vi "App - RUS scan.vi"(0 "Lock-in DAQ settings":T5={"Lockin mode"=enum."NI-DAQ", "DAQmx Device"="Dev1", "SR Lockin"="GPIB0::10::INSTR", "Clock Multiplier"=64, "Low-pass filter"=enum."No filtering", "Ranges and couplings "=[{"Range"=2.5, "Coupling"=10106}], "Samples per read"=20, "Record IF"=FALSE, "Auto-phase"=FALSE, "RP IP Addres"="172.20.117.190"} {"Ranges and couplings"."Coupling" items=["default"=-1, "RSE"=10083, "NRSE"=10078, "Differential"=10106, "Pseudodifferential"=12529]}, 1 "Save data settings":T7={"Save data"=TRUE, "Data Root Path"=path "E:/Technique/RUS/Saphire/Saphire_piece1/1_test", "File Prefix"="291.30300K_2000_3000_2.00000V_0.00000T_Jul26-2016__14-58-15_", "File Format"=enum."BINARY", "Save column names"=FALSE, "File Comments"="\r\nColumns:Frequency\\tX\\tY\r\n    ITC Temp= 299.200000\r\n    LTC Temp= 0.000000\r\n          ITC_set=295.00000\r\n", "User/Prj"="<User Name/Project Description>"}, 5 "temperature":dbl=291.303, 7 "sweep settings":T1={"time gap (min) "=0.0, "Bypass error dialog"=TRUE, "range factor"=1.2, "min gamma(kHz)"=0.005, "max step(Hz)"=1500.0, "min step(Hz)"=0.001, "save freq units"=enum."kHz", "Zero signal?"=FALSE, "time in Gamma --OK"=FALSE, "scan mode"=enum."uniform", "power control mode "=enum."none", "time-in-gamma mode"=enum."uniform scan"}, 9 "Fast swep settings":T4={"Update rate (Hz)"=200.0, "Start F, Hz"=2000000.0, "Stop F"=3000000.0, "Number of points"=5760, "Amplitude"=2.0, "Init&amplitude"=TRUE, "IF"=1000.0, "Time constant"=0.0042} {"IF" format="%#_6p"; "Amplitude" min=0.0 max=2.5; "Number of points" format="%.0p"; "Stop F" format="%#_6p"; "Start F, Hz" format="%#_6p"; "Update rate (Hz)" format="%0.2f"}, 11 "error in (no error)":errorcluster) -> (6 "Actual file path":path=path "E:/Technique/RUS/Saphire/Saphire_piece1/1_test/July_2016/072616/291.31700K_2000_3000_2.00000V_0.00000T_Jul26-2016__14-57-42_001_072616.bin", 15 "error out":errorcluster)   [LabVIEW 2016]
uses:
  <vilib>/Utility/error.llb/DialogType.ctl
  <resource>/objmgr/daqmx.rc
  next chunk -- action.ctl
  cursor action.ctl
  four-corner circle transformation.ctl
  circle corners.ctl
  NHMFL_Core/Libraries/Red Pitaya/RP Core/RP Transceiver/RP Transceiver.lvclass
  resonant_ultrasound/Libraries/RUS/Controls/Sweep settings.ctl
  resonant_ultrasound/Libraries/RUS/Controls/Lock-in DAQ settings.ctl
  NHMFL_Core/Libraries/File/Controls/File formats.ctl
  NHMFL_Core/Libraries/File/Controls/Save data settings.ctl
  single sweep - adaptive parameters.ctl
  single sweep - frequency chunks.ctl
  wavepacket.ctl
  next chunk -- parameters.ctl
  next chunk -- algorithm.ctl
  find peak -- parameters.ctl
  adaptive sweep UI controls.ctl
  time in gamma mode control.ctl
  resonant_ultrasound/Libraries/RUS/Controls/Lockin mode.ctl
panel:
  in  "Tab : everything":enum32{"main", "everything else", "adaptive"}(tab)
  out "near omega (kHz)":dbl
  in  "Subtract a circle?":enum16{"Yes", "No"}(ring)=enum."No"
  in  "complex plane scale gauge":dbl(slide)=0.012396748308571648 caption="Volts" scale=0.0001..0.5
  in  "show plot pallets":bool=TRUE
  in  "highlight last # sec":dbl=5.0
  out "Plot:response":cluster{dbl[], dbl[]}[](graph)=[{array[5760 elements], array[960 elements]}, {array[5760 elements], array[960 elements]}, {[2225.33441, 2225.33441], [-0.001, 0.001]}, {[3002.8544, 3002.8544], [-0.001, 0.001]}, {[4313.39901, 4313.39901], [-0.001, 0.001]}, {[4368.99077, 4368.99077], [-0.001, 0.001]}, {[5103.78232, 5103.78232], [-0.001, 0.001]}, {[5322.11972, 5322.11972], [-0.001, 0.001]}, {[5780.98612, 5780.98612], [-0.001, 0.001]}, {[6352.47126, 6352.47126], [-0.001, 0.001]}]
  out "Plot:complex plane":cluster{dbl[], dbl[]}[](graph)=[{array[960 elements], array[960 elements]}, {array[1000 elements], array[1000 elements]}, {[0.005000003045536789, 0.004940547817909086, 0.004763119779482496, 0.004470517076413378, 0.004067354228121515, 0.0035599893535622827, 0.0029564238998925634, 0.0022661764548692546, 0.0015001326330342118, 0.0006703734030701707, -0.00021001543629219814, -0.0011271496271373508, -0.0020665654154062474, -0.003013447652938098, -0.003952863441206996, -0.004869997632052148, -0.005750386471414516, -0.0065801457013785584, -0.0073461895232136, -0.008036436968236908, -0.008640002421906627, -0.009147367296465859, -0.009550530144757723, -0.00984313284782684, -0.010020560886253431, -0.010080016113881134, -0.010020560886253431, -0.00984313284782684, -0.009550530144757721, -0.009147367296465859, -0.008640002421906625, -0.008036436968236908, -0.007346189523213599, -0.006580145701378555, -0.005750386471414511, -0.004869997632052148, -0.003952863441206995, -0.0030134476529380966, -0.0020665654154062444, -0.0011271496271373462, -0.00021001543629219988, 0.0006703734030701703, 0.0015001326330342135, 0.0022661764548692572, 0.002956423899892566, 0.0035599893535622853, 0.004067354228121515, 0.004470517076413378, 0.004763119779482496, 0.004940547817909086], [0.00047076259399639255, 0.0014157763757271474, 0.0023458867255961384, 0.0032464252477649408, 0.004103189911783316, 0.004902669027093289, 0.0056322543304607505, 0.00628043982581846, 0.006837003240697381, 0.007293167237570003, 0.007641737837706482, 0.007877217874516685, 0.007995893687151154, 0.007995893687151154, 0.007877217874516684, 0.007641737837706482, 0.0072931672375700024, 0.00683700324069738, 0.00628043982581846, 0.005632254330460749, 0.0049026690270932895, 0.004103189911783315, 0.003246425247764939, 0.002345886725596139, 0.0014157763757271461, 0.0004707625939963901, -0.00047425118773436253, -0.0014043615376033549, -0.0023049000597721585, -0.0031616647237905308, -0.0039611438391005055, -0.004690729142467966, -0.005338914637825676, -0.005895478052704598, -0.00635164204957722, -0.0067002126497136974, -0.0069356926865239, -0.007054368499158369, -0.007054368499158369, -0.006935692686523899, -0.006700212649713698, -0.006351642049577218, -0.005895478052704595, -0.0053389146378256735, -0.004690729142467962, -0.0039611438391004995, -0.0031616647237905303, -0.002304900059772155, -0.001404361537603351, -0.00047425118773435874]}, {[-0.0036773228927567273, -0.003563591256898272, -0.0034498596210398164, -0.003336127985181361, -0.0032223963493229054, -0.0031086647134644495, -0.0029949330776059945, -0.0028812014417475386, -0.002767469805889083, -0.0026537381700306277, -0.0025400065341721722, -0.0024262748983137168, -0.0023125432624552613, -0.002198811626596806, -0.00208507999073835, -0.001971348354879895, -0.0018576167190214393, -0.0017438850831629838, -0.0016301534473045281, -0.0015164218114460727], [0.00792450366560593, 0.007179129558444975, 0.006433755451284022, 0.005688381344123069, 0.004943007236962115, 0.004197633129801161, 0.0034522590226402083, 0.0027068849154792546, 0.001961510808318301, 0.001216136701157347, 0.0004707625939963933, -0.00027461151316456045, -0.0010199856203255125, -0.0017653597274864662, -0.00251073383464742, -0.0032561079418083737, -0.0040014820489693275, -0.004746856156130281, -0.005492230263291235, -0.006237604370452189]}, {[0.004913734537437363, 0.004168360430276409, 0.003422986323115456, 0.0026776122159545028, 0.001932238108793549, 0.0011868640016325952, 0.00044148989447164236, -0.0003038842126893114, -0.0010492583198502652, -0.001794632427011219, -0.0025400065341721727, -0.0032853806413331264, -0.0040307547484940785, -0.004776128855655032, -0.005521502962815986, -0.00626687706997694, -0.0070122511771378935, -0.007757625284298847, -0.008502999391459801, -0.009248373498620755], [0.0016080789525809475, 0.001494347316722492, 0.0013806156808640366, 0.001266884045005581, 0.0011531524091471254, 0.00103942077328867, 0.0009256891374302145, 0.0008119575015717589, 0.0006982258657133035, 0.0005844942298548479, 0.00047076259399639244, 0.000357030958137937, 0.00024329932227948152, 0.00012956768642102606, 1.5836050562570382e-05, -9.789558529588508e-05, -0.00021162722115434054, -0.000325358857012796, -0.0004390904928712517, -0.0005528221287297071]}]
  in  "progress (sec)":dbl(slide)=4.701000000000931 caption="seconds" min=80.0 max=80.0 scale=0.0..28.8
  in  "Plot when running":bool=TRUE
  in  "Graph update rate, ms":u32=50
  out "near gamma (kHz)":dbl
  in  "stop":bool
  out "Progress, %":u8(slide)=16 scale=0.0..100.0
  in  "Tab : sweep controls":enum32{"Main controls", "File", "Advanced"}(tab)
  in  "Manual\nPhase":dbl(slide) scale=-180.0..180.0
  out "Error status byte\n(bit 5 - FAST aborted)":u8 format="%08b"
  out "STD status byte":u8 format="%08b"
  out "DO array  making time":u32
  out "DO write time, ms":u32=37
  out "Loop counter":i32=287
  out "Pre-sweep delay, s":dbl=0.2
  out "Samples in buffer":u32
  out "Actual setup time, ms":u32=2842
  out "line two":cluster{dbl[], dbl[]}={[0.004913734537437363, 0.004168360430276409, 0.003422986323115456, 0.0026776122159545028, 0.001932238108793549, 0.0011868640016325952, 0.00044148989447164236, -0.0003038842126893114, -0.0010492583198502652, -0.001794632427011219, -0.0025400065341721727, -0.0032853806413331264, -0.0040307547484940785, -0.004776128855655032, -0.005521502962815986, -0.00626687706997694, -0.0070122511771378935, -0.007757625284298847, -0.008502999391459801, -0.009248373498620755], [0.0016080789525809475, 0.001494347316722492, 0.0013806156808640366, 0.001266884045005581, 0.0011531524091471254, 0.00103942077328867, 0.0009256891374302145, 0.0008119575015717589, 0.0006982258657133035, 0.0005844942298548479, 0.00047076259399639244, 0.000357030958137937, 0.00024329932227948152, 0.00012956768642102606, 1.5836050562570382e-05, -9.789558529588508e-05, -0.00021162722115434054, -0.000325358857012796, -0.0004390904928712517, -0.0005528221287297071]}
  out "circle":cluster{dbl[], dbl[]}={[0.005000003045536789, 0.004940547817909086, 0.004763119779482496, 0.004470517076413378, 0.004067354228121515, 0.0035599893535622827, 0.0029564238998925634, 0.0022661764548692546, 0.0015001326330342118, 0.0006703734030701707, -0.00021001543629219814, -0.0011271496271373508, -0.0020665654154062474, -0.003013447652938098, -0.003952863441206996, -0.004869997632052148, -0.005750386471414516, -0.0065801457013785584, -0.0073461895232136, -0.008036436968236908, -0.008640002421906627, -0.009147367296465859, -0.009550530144757723, -0.00984313284782684, -0.010020560886253431, -0.010080016113881134, -0.010020560886253431, -0.00984313284782684, -0.009550530144757721, -0.009147367296465859, -0.008640002421906625, -0.008036436968236908, -0.007346189523213599, -0.006580145701378555, -0.005750386471414511, -0.004869997632052148, -0.003952863441206995, -0.0030134476529380966, -0.0020665654154062444, -0.0011271496271373462, -0.00021001543629219988, 0.0006703734030701703, 0.0015001326330342135, 0.0022661764548692572, 0.002956423899892566, 0.0035599893535622853, 0.004067354228121515, 0.004470517076413378, 0.004763119779482496, 0.004940547817909086], [0.00047076259399639255, 0.0014157763757271474, 0.0023458867255961384, 0.0032464252477649408, 0.004103189911783316, 0.004902669027093289, 0.0056322543304607505, 0.00628043982581846, 0.006837003240697381, 0.007293167237570003, 0.007641737837706482, 0.007877217874516685, 0.007995893687151154, 0.007995893687151154, 0.007877217874516684, 0.007641737837706482, 0.0072931672375700024, 0.00683700324069738, 0.00628043982581846, 0.005632254330460749, 0.0049026690270932895, 0.004103189911783315, 0.003246425247764939, 0.002345886725596139, 0.0014157763757271461, 0.0004707625939963901, -0.00047425118773436253, -0.0014043615376033549, -0.0023049000597721585, -0.0031616647237905308, -0.0039611438391005055, -0.004690729142467966, -0.005338914637825676, -0.005895478052704598, -0.00635164204957722, -0.0067002126497136974, -0.0069356926865239, -0.007054368499158369, -0.007054368499158369, -0.006935692686523899, -0.006700212649713698, -0.006351642049577218, -0.005895478052704595, -0.0053389146378256735, -0.004690729142467962, -0.0039611438391004995, -0.0031616647237905303, -0.002304900059772155, -0.001404361537603351, -0.00047425118773435874]}
  out "line one":cluster{dbl[], dbl[]}={[-0.0036773228927567273, -0.003563591256898272, -0.0034498596210398164, -0.003336127985181361, -0.0032223963493229054, -0.0031086647134644495, -0.0029949330776059945, -0.0028812014417475386, -0.002767469805889083, -0.0026537381700306277, -0.0025400065341721722, -0.0024262748983137168, -0.0023125432624552613, -0.002198811626596806, -0.00208507999073835, -0.001971348354879895, -0.0018576167190214393, -0.0017438850831629838, -0.0016301534473045281, -0.0015164218114460727], [0.00792450366560593, 0.007179129558444975, 0.006433755451284022, 0.005688381344123069, 0.004943007236962115, 0.004197633129801161, 0.0034522590226402083, 0.0027068849154792546, 0.001961510808318301, 0.001216136701157347, 0.0004707625939963933, -0.00027461151316456045, -0.0010199856203255125, -0.0017653597274864662, -0.00251073383464742, -0.0032561079418083737, -0.0040014820489693275, -0.004746856156130281, -0.005492230263291235, -0.006237604370452189]}
  out "frequency":dbl[](array[numeric])
  out "complex data":cdb[](array[numeric])
  out "#data points so far":i32=960
  out "last data":cdb[](array[numeric])=[-1.8863502679099892e-05+1.1101912486449137e-05i, -1.3771240984552797e-05+1.353770104896233e-05i, 8.815893688967333e-06-8.669622050274321e-07i, 4.353149549589407e-06-5.242292389749474e-06i, -2.0188892981734304e-05+2.69270732421671e-06i, -3.236472954490424e-05-1.4037098105498458e-05i, -1.4486448565831475e-06+5.6829496403972965e-06i, 2.1749189330097788e-05-2.2323271152381018e-05i, 1.0947860915724242e-05-9.35400417253664e-06i, 1.002480840777342e-06+1.0320450470074709e-05i, 1.7405541793727768e-05+1.8150037416439624e-05i, -3.440648475476081e-06-3.0319378431607727e-06i, -5.515652282118088e-06+8.369787998015825e-06i, 1.3508753228977962e-06-9.402754381312778e-07i, -9.163410786339015e-06+3.1872150390602785e-05i, 1.843763405159508e-05+9.77165232492216e-07i, 1.6194427097054223e-05+8.11657185157076e-06i, -1.892640018440827e-05+1.3227915471368098e-05i, -1.8081522602619296e-05+1.6532235062315973e-05i, 1.084682936928357e-05+3.944687906764937e-06i]
  out "fancy circles":cluster{dbl[], dbl[]}[](array[cluster])
  out "fancy lines":cluster{dbl[], dbl[]}[](array[cluster])=[{[2225.33441, 2225.33441], [-0.001, 0.001]}, {[3002.8544, 3002.8544], [-0.001, 0.001]}, {[4313.39901, 4313.39901], [-0.001, 0.001]}, {[4368.99077, 4368.99077], [-0.001, 0.001]}, {[5103.78232, 5103.78232], [-0.001, 0.001]}, {[5322.11972, 5322.11972], [-0.001, 0.001]}, {[5780.98612, 5780.98612], [-0.001, 0.001]}, {[6352.47126, 6352.47126], [-0.001, 0.001]}]
  in  "adaptive state":T9={"peaks are known -- parameters"={"Def Gamma (kHz)"=10.0, "dV"=17.0, "time in Gamma (sec)"=3.0, "phi-star"=0.0, "all peaks (kHz)"=[2225.33441, 3002.8544, 4313.39901, 4368.99077, 5103.78232, 5322.11972, 5780.98612, 6352.47126], "delta t (sec)"=0.005, "default step (Hz)"=173.61111111111111, "all gamma (kHz)"=[0.92069, 0.9684, 1.01783, 0.32516, 1.96607, 0.61241, 0.19018, 0.73869], "peaks OK"=TRUE, "gamma OK"=TRUE, "near omega (kHz)"=0.0, "near gamma (kHz)"=0.0, "min step (Hz)"=0.001, "max step(Hz)"=1500.0, "min gamma (kHz)"=0.005, "all time in gamma (sec)"=[], "time in gamma OK"=FALSE, "time-in-gamma mode"=enum."same for all"}, "find peak - parameters"={"wavepacket"={"R"=0.5, "wave number"=17.0, "delta k"=7.0, "radii vector"=[], "radial section"=[], "wave vector"=22.0, "wavepacket is"=TRUE}, "number of grid points"=70, "decimation threshold"=1, "Voltage range"=0.1, "target freq step"=20.0, "target spot size"=0.05, "factor"=1.0, "another factor"=1.0, "analyze last # sec"=3, "scale factor"=3}} {"find peak - parameters"."wavepacket"."delta k" format="%#_3f"; "find peak - parameters"."wavepacket"."wave number" format="%#_3f"; "find peak - parameters"."wavepacket"."R" format="%#_3f"}
  in  "chunks":T13={"start F (Hz)"=2000000.0, "stop F (Hz)"=3000000.0, "total number of points"=5760, "chunk size"=20, "freq step (Hz)"=173.61111111111111, "update rate (Hz)"=200.0, "adaptive parameters"={"peaks are known -- parameters"={"Def Gamma (kHz)"=10.0, "dV"=17.0, "time in Gamma (sec)"=3.0, "phi-star"=0.0, "all peaks (kHz)"=[2225.33441, 3002.8544, 4313.39901, 4368.99077, 5103.78232, 5322.11972, 5780.98612, 6352.47126], "delta t (sec)"=0.005, "default step (Hz)"=173.61111111111111, "all gamma (kHz)"=[0.92069, 0.9684, 1.01783, 0.32516, 1.96607, 0.61241, 0.19018, 0.73869], "peaks OK"=TRUE, "gamma OK"=TRUE, "near omega (kHz)"=0.0, "near gamma (kHz)"=0.0, "min step (Hz)"=0.001, "max step(Hz)"=1500.0, "min gamma (kHz)"=0.005, "all time in gamma (sec)"=[], "time in gamma OK"=FALSE, "time-in-gamma mode"=enum."same for all"}, "find peak - parameters"={"wavepacket"={"R"=0.5, "wave number"=17.0, "delta k"=7.0, "radii vector"=[], "radial section"=[], "wave vector"=22.0, "wavepacket is"=TRUE}, "number of grid points"=70, "decimation threshold"=1, "Voltage range"=0.1, "target freq step"=20.0, "target spot size"=0.05, "factor"=1.0, "another factor"=1.0, "analyze last # sec"=3, "scale factor"=3}}, "total sweep time (sec)"=28.8, "chunk time (sec)"=0.1, "spot size (V)"=0.0, "uniform freq step (Hz)"=173.61111111111111, "next start freq (Hz)"=2177083.3333333293} {"next start freq (Hz)" format="%#9_8f"; "uniform freq step (Hz)" format="%#_3f"; "spot size (V)" format="%#_2f"; "adaptive parameters"."find peak - parameters"."wavepacket"."delta k" format="%#_3f"; "adaptive parameters"."find peak - parameters"."wavepacket"."wave number" format="%#_3f"; "adaptive parameters"."find peak - parameters"."wavepacket"."R" format="%#_3f"; "freq step (Hz)" format="%#4_4f"; "stop F (Hz)" format="%#_3f"; "start F (Hz)" format="%#_3f"}
  # "SRS Lockin related"
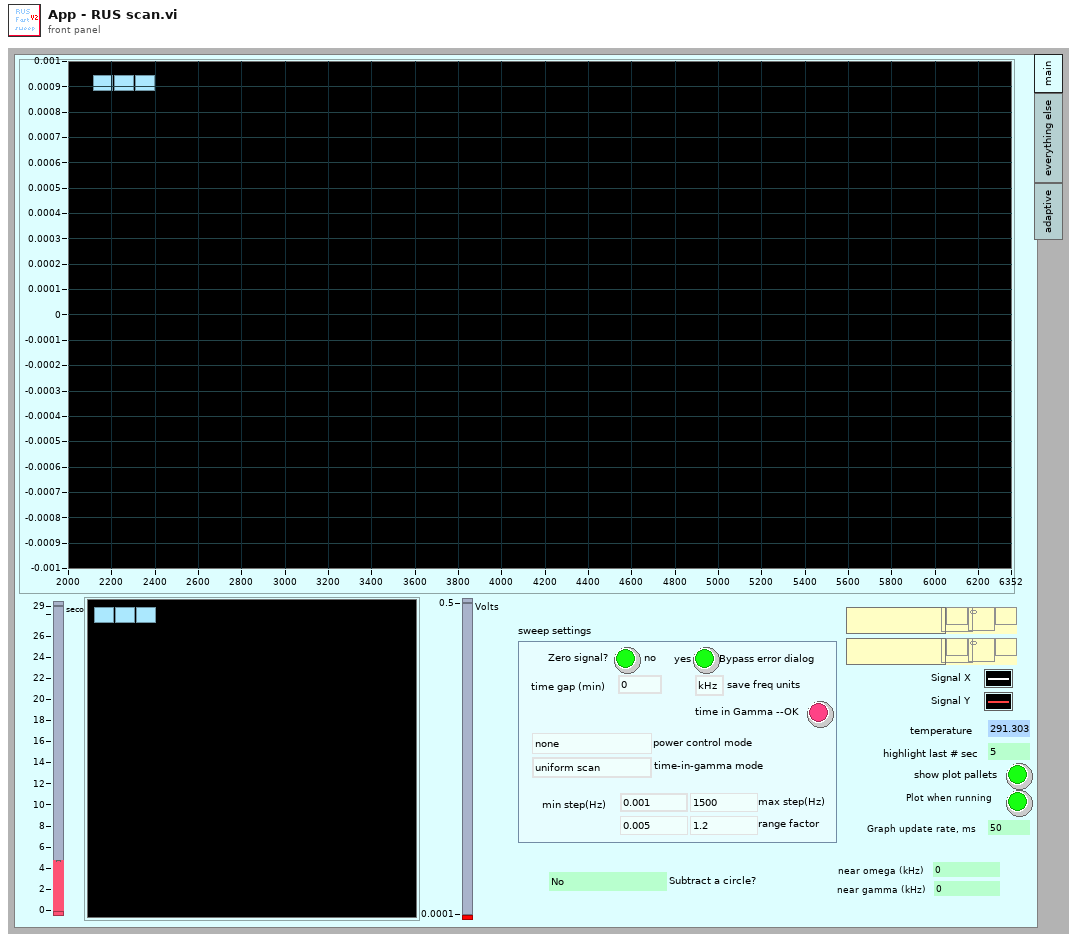
[diagram p1: front panel]
types:
  T1 = typedef "adaptive sweep UI controls.ctl" = cluster{"time gap (min) ":dbl, "Bypass error dialog":bool, "range factor":dbl, "min gamma(kHz)":dbl, "max step(Hz)":dbl, "min step(Hz)":dbl, "save freq units":enum16{"kHz", "Hz"}, "Zero signal?":bool, "time in Gamma --OK":bool, "scan mode":T2, "power control mode ":enum16{"power vs Temp", "power vs Time", "none"}, "time-in-gamma mode":T3}
  T2 = typedef "next chunk -- algorithm.ctl" = enum16{"peak position is known", "uniform", "predictive"}
  T3 = typedef "time in gamma mode control.ctl" = enum16{"same for all", "each one different", "uniform scan"}
  T4 = typedef "Sweep settings.ctl" = cluster{"Update rate (Hz)":dbl, "Start F, Hz":dbl, "Stop F":dbl, "Number of points":i32, "Amplitude":dbl, "Init&amplitude":bool, "IF":dbl, "Time constant":dbl}
  T5 = typedef "Lock-in DAQ settings.ctl" = cluster{"Lockin mode":T6, "DAQmx Device":tag, "SR Lockin":refnum<visa-resource-name>, "Clock Multiplier":i32, "Low-pass filter":enum16{"No filtering", "Butterworth", "Bessel"}, "Ranges and couplings ":cluster{"Range":dbl, "Coupling":i32}[], "Samples per read":i32, "Record IF":bool, "Auto-phase":bool, "RP IP Addres":string}
  T6 = typedef "Lockin mode.ctl" = enum16{"SRS", "NI-DAQ", "Pitaya"}
  T7 = typedef "Save data settings.ctl" = cluster{"Save data":bool, "Data Root Path":path, "File Prefix":string, "File Format":T8, "Save column names":bool, "File Comments":string, "User/Prj":string}
  T8 = typedef "File formats.ctl" = enum16{"TDMS", "ASCII", "BINARY"}
  T9 = typedef "single sweep - adaptive parameters.ctl" = cluster{"peaks are known -- parameters":T10, "find peak - parameters":T11}
  T10 = typedef "next chunk -- parameters.ctl" = cluster{"Def Gamma (kHz)":dbl, "dV":dbl, "time in Gamma (sec)":dbl, "phi-star":dbl, "all peaks (kHz)":dbl[], "delta t (sec)":dbl, "default step (Hz)":dbl, "all gamma (kHz)":dbl[], "peaks OK":bool, "gamma OK":bool, "near omega (kHz)":dbl, "near gamma (kHz)":dbl, "min step (Hz)":dbl, "max step(Hz)":dbl, "min gamma (kHz)":dbl, "all time in gamma (sec)":dbl[], "time in gamma OK":bool, "time-in-gamma mode":T3}
  T11 = typedef "find peak -- parameters.ctl" = cluster{"wavepacket":T12, "number of grid points":i32, "decimation threshold":i32, "Voltage range":dbl, "target freq step":dbl, "target spot size":dbl, "factor":dbl, "another factor":dbl, "analyze last # sec":i32, "scale factor":i32}
  T12 = typedef "wavepacket.ctl" = cluster{"R":dbl, "wave number":dbl, "delta k":dbl, "radii vector":dbl[], "radial section":cdb[], "wave vector":dbl, "wavepacket is":bool}
  T13 = typedef "single sweep - frequency chunks.ctl" = cluster{"start F (Hz)":dbl, "stop F (Hz)":dbl, "total number of points":i32, "chunk size":i32, "freq step (Hz)":dbl, "update rate (Hz)":dbl, "adaptive parameters":T9, "total sweep time (sec)":dbl, "chunk time (sec)":dbl, "spot size (V)":dbl, "uniform freq step (Hz)":dbl, "next start freq (Hz)":dbl}
  T14 = typedef "RUS settings.ctl" = cluster{"NI-DAQ lockin settings":T15, "Fast swep settings":T4, "Pre-sweep delay, s":dbl, "Lockin mode":T6, "SR Lockin":refnum<visa-resource-name>, "DAQmx Device":tag, "Clock Multiplier":i32, "Fast Sweep Data Out":cluster{"DO clock task":refnum<k21>, "DO task":refnum<k21>, "Update clock task":refnum<k21>, "DAQ lockin task":refnum<k21>, "Pre-sweep counter task":refnum<k21>}, "Lockin Range, V":sgl, "F Array":dbl[], "Freq. update clock terminal":string, "DO Clock Rate (Hz)":dbl, "ADC clock terminal":string, "Pre-sweep counter terminal":string, "Samples per read":i32, "DO clock terminal":string, "Pre-sweep points":i32, "F points per write":i32, "Total sweep time, s":dbl, "Initial SYNTH phase":dbl, "Record IF":bool, "Save data settings":T7, "Data file path":path, "New data user event":refnum<user-event>, "Stop user event":refnum<user-event>, "Number of channels":i32, "Auto-phase":bool, "RP Transeiver":refnum<class "RP Transceiver.lvclass">}
  T15 = typedef "RUS NI-DAQ Lockin Settings.ctl" = cluster{"Samples per sine wave":i32, "Sine waves per freq step":i32, "Output Representation":enum16{"Real/Imaginary", "Polar"}, "Low-pass filter":enum16{"No filtering", "Butterworth", "Bessel"}, "Ranges and couplings ":cluster{"Range":dbl, "Coupling":i32}[]}
  T16 = typedef "next chunk -- action.ctl" = enum16{"empty", "init - uniform", "next chunk - uniform", "next chunk - peaks are known", "init - peaks are known", ""}
  T17 = typedef "circle corners.ctl" = cluster{"z (-pi/2)":cdb, "z(inf)":cdb, "z (pi/2)":cdb, "z center":cdb, "z(0)":cdb, "radius":dbl}
  T18 = typedef "four-corner circle transformation.ctl" = enum16{"z(c) z(inf)", "z(c) z(zero)", "fix phase", "calculate lorentzian", "z(0) z(+-pi/2)", "shift to zcenter"}
  T19 = typedef "cursor action.ctl" = enum16{"range", "read", "write", "check", "zoom out", "smart zoom out"}
  T20 = typedef "DialogType.ctl" = u16
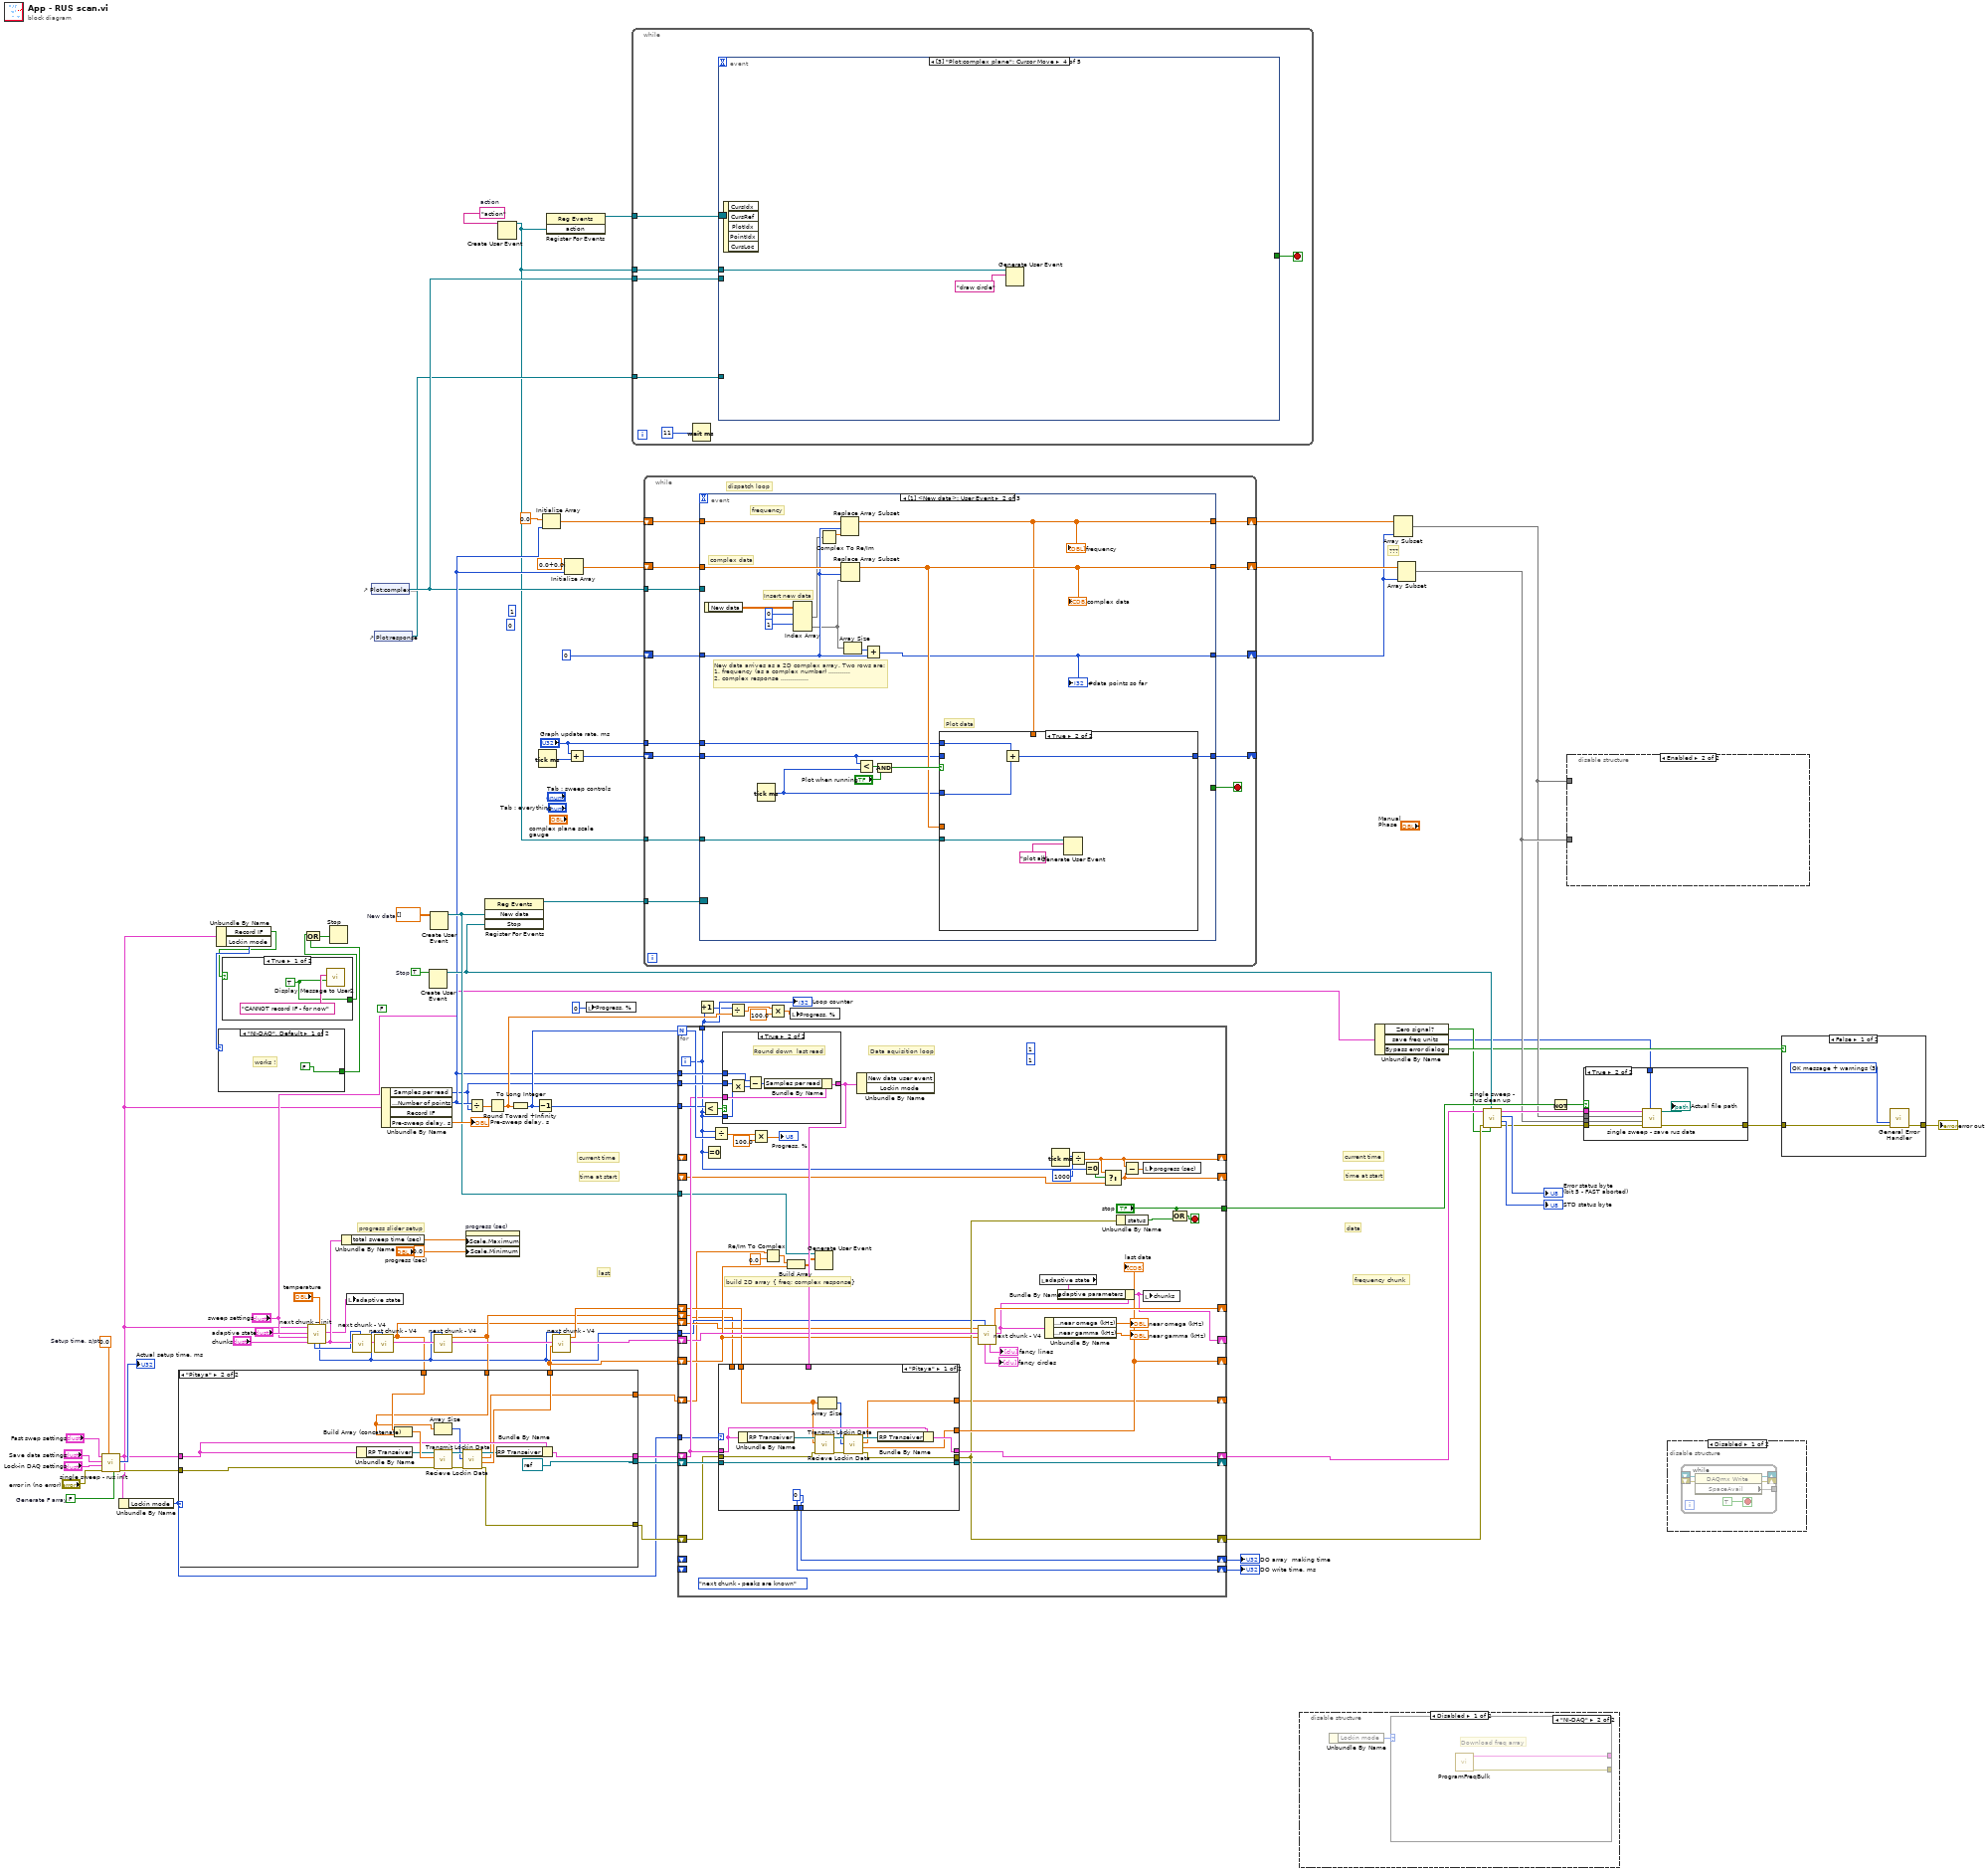
[diagram p0: block diagram]
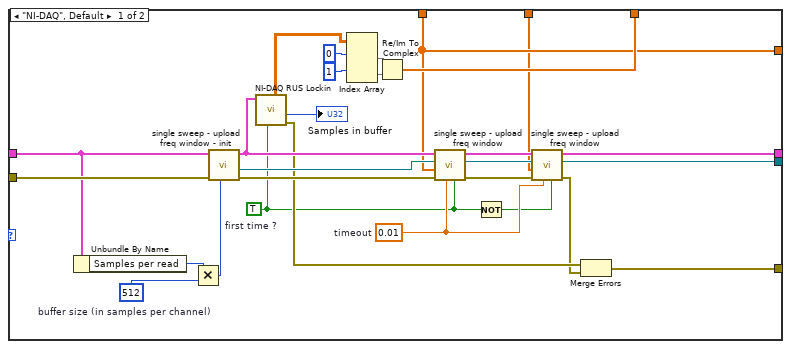
[diagram p2: hidden frame]
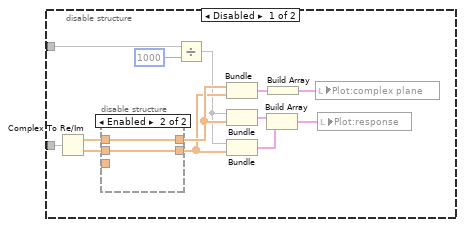
[diagram p3: hidden frame]
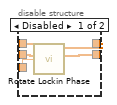
[diagram p4: hidden frame]
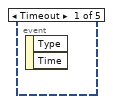
[diagram p5: hidden frame]
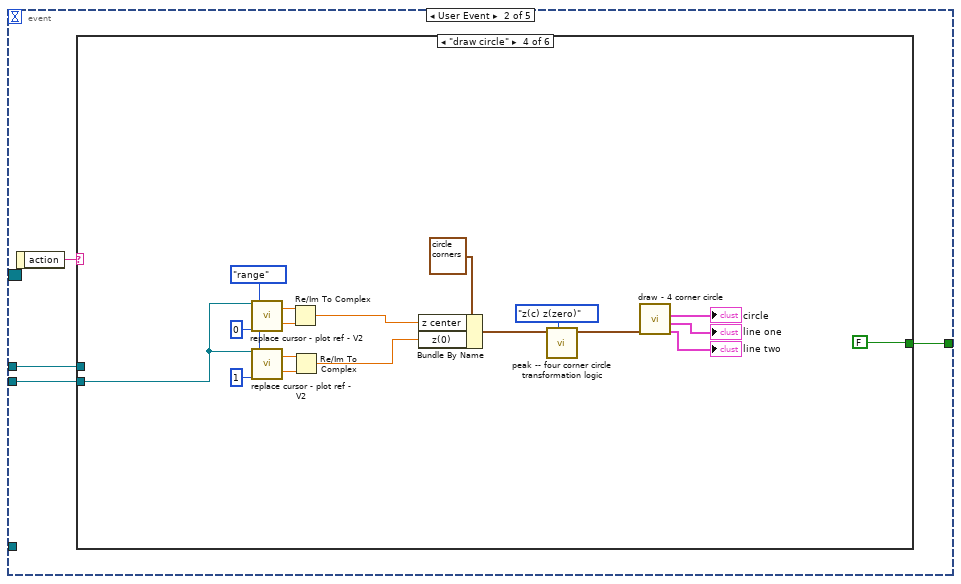
[diagram p6: hidden frame]
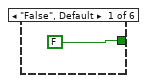
[diagram p7: hidden frame]
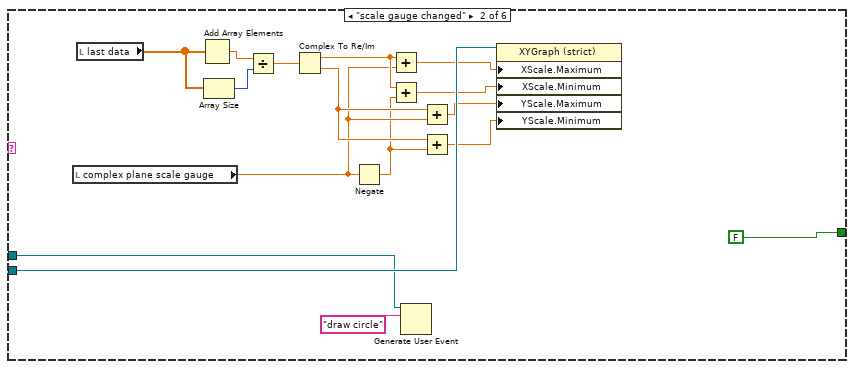
[diagram p8: hidden frame]
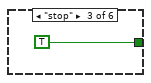
[diagram p9: hidden frame]
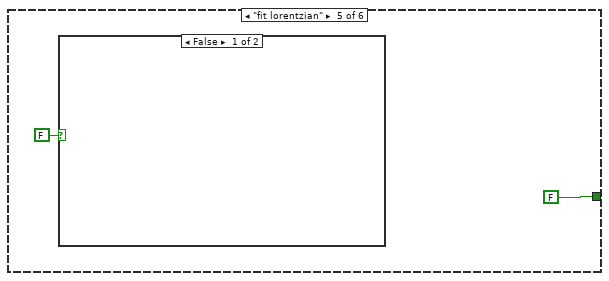
[diagram p10: hidden frame]
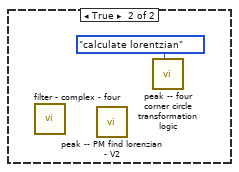
[diagram p11: hidden frame]
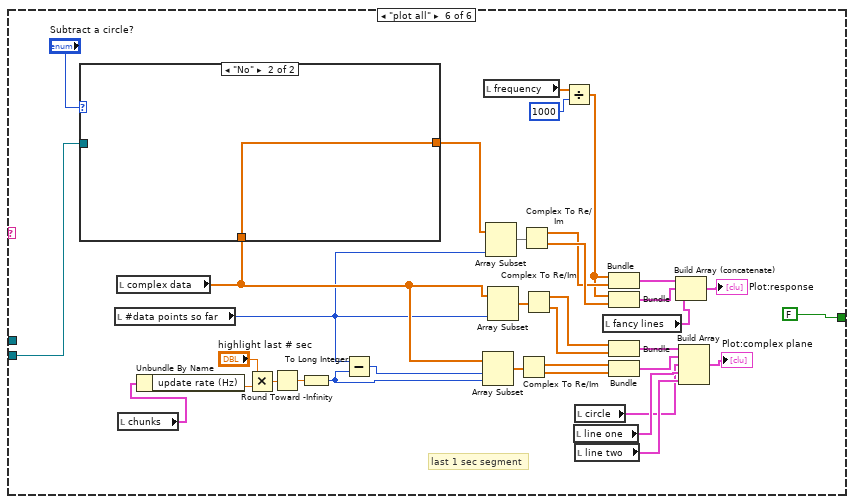
[diagram p12: hidden frame]
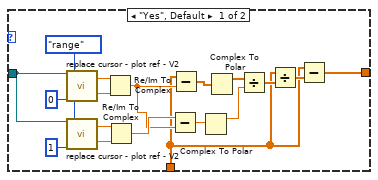
[diagram p13: hidden frame]
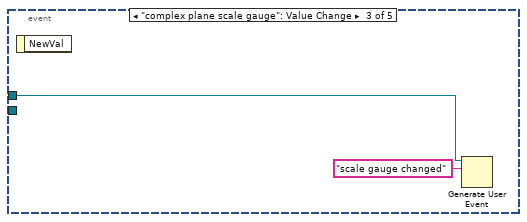
[diagram p14: hidden frame]
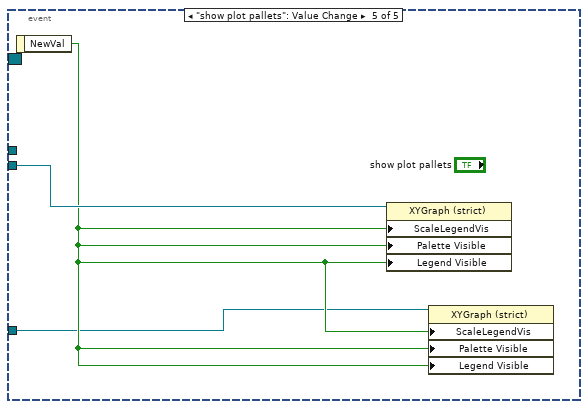
[diagram p15: hidden frame]
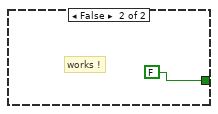
[diagram p17: hidden frame]
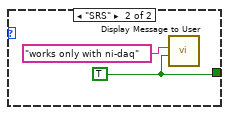
[diagram p18: hidden frame]
diagram:
  w8 = "action"  # action
  w22 = FALSE  # Generate F array
  w23 = 0.0  # Setup time, s/pt
  (unwired) 0 ("disabled index (col)")
  (unwired) FALSE
  (unwired) 1 ("dimension size")
  w50 = cdb[][] []  # New data
  w52 = TRUE  # Stop
  # "data"
  # "frequency chunk"
  # "last"
  # "time at start"
  # "current time"
  # "time at start"
  # "current time"
  # "progress slider setup"
  # "???"
  n1 = call "single sweep - rus init.vi"("Generate F array"=w22, "Setup time, s/pt"=w23, "error in (no error)"="error in (no error)", "Lock-in DAQ settings"="Lock-in DAQ settings", "Save data settings"="Save data settings", "Fast swep settings"="Fast swep settings") -> ("error out"=w57:errorcluster, "Actual setup time, ms"=→"Actual setup time, ms":u32, "RUS settings out"=w3:T14)  [unwired: 2 in, 1 out]
  n2 = Unbundle By Name(w3) -> ("Lockin mode"=w1:T6)
  n3 = Unbundle By Name(w3) -> ("Record IF"=w39:bool, "Lockin mode"=w56:T6)
  n4 = case shown="\"NI-DAQ\", Default" w56 {
    tunnel: [FALSE w89] -> w41
    frame "NI-DAQ", Default {
      # "works !"
    }
    frame "SRS" {
      w89 = TRUE
      n5 = call "Display Message to User"("Enable"=w89, "Message"="works only with ni-daq") -> ()  [unwired: 8 in, 2 out]
    }
  }
  n6 = case shown="True" w39 {
    tunnel: [w91 FALSE] -> w40
    frame True {
      w91 = TRUE
      n7 = call "Display Message to User2"("Enable"=w91, "Message"="CANNOT record IF - for now") -> ()  [unwired: 8 in, 2 out]
    }
    frame False {
      # "works !"
    }
  }
  n8 = Or(x=w40, y=w41) -> (x .or. y?=w38:bool)
  n9 = call "next chunk -- init.vi"("temperature"="temperature", "chunks"="chunks", "sweep settings"="sweep settings", "adaptive parameters"="adaptive state", "RUS settings"=w3) -> ("chunks out"=w20:T13, "adaptive parameters out"=w18:T9, "next chunk action"=w14:T16, "next chunk init action"=w17:T16)  [unwired: 3 in]
  n10 = Stop(stop? (T)=w38) -> ()
  n11 = Unbundle By Name(w20) -> ("total sweep time (sec)"=w37:dbl)
  n12 = local write "adaptive state"(w18) -> ()
  n13 = call "next chunk - V4.vi"("next chunk action"=w17, "chunks"=w20) -> ("chunks out"=w15:T13)  [unwired: 6 in, 3 out]
  n14 = control-ref of="Plot:complex plane"() -> (w6:refnum<vi>)
  n15 = control-ref of="Plot:response"() -> (w5:refnum<vi>)
  n16 = call "next chunk - V4.vi"("next chunk action"=w14, "chunks"=w15) -> ("F Array out"=w13:dbl[])  [unwired: 6 in, 3 out]
  n17 = Unbundle By Name(w3) -> ("Samples per read"=w33:i32, "Fast swep settings.Number of points"=w34:i32, "Pre-sweep delay, s"=→"Pre-sweep delay, s":dbl)  [unwired: 1 out]
  n18 = Create User Event(user event datatype=w52) -> (user event=w45:refnum<user-event>)  [unwired: 1 in, 1 out]
  n19 = Create User Event(user event datatype=w50) -> (user event=w51:refnum<user-event>)  [unwired: 1 in, 1 out]
  n20 = call "next chunk - V4.vi"("next chunk action"=w14, "chunks"=w15) -> ("chunks out"=w30:T13, "F Array out"=w24:dbl[])  [unwired: 6 in, 2 out]
  n21 = case shown="\"Pitaya\"" w1 {
    tunnel: w57 -> [w121 w131]
    tunnel: [w117 w127] -> w32
    tunnel: [w116 refnum<k21> refnum ("task out")] -> w31
    tunnel: [w113 w125] -> w28
    tunnel: [w110 w128] -> w25
    tunnel: w24 -> [w94 w123]
    tunnel: w3 -> [w98 w133]
    tunnel: w13 -> [w95 w135]
    tunnel: [w95 w124] -> w2
    frame "NI-DAQ", Default {
      w96 = TRUE  # first time ?
      w109 = u32 512  # buffer size (in samples per channel)
      w114 = 0.01  # timeout
      n22 = Unbundle By Name(w98) -> ("Samples per read"=w107:i32)
      n23 = Multiply(x=w107, y=w109) -> (x*y=w108:u32)
      n24 = call "single sweep - upload freq window - init.vi"("buffer size (in samples per channel)"=w108, "error in (no error)"=w121, "RUS settings"=w98) -> ("error - out"=w112:errorcluster, "task out"=w120:refnum<k21>, "RUS settings out"=w119:T14)  [unwired: 6 in]
      n25 = call "NI-DAQ RUS Lockin.vi"("Init?"=w96, "RUS settings"=w119) -> ("error out"=w100:errorcluster, "AvailSampPerChan"=→"Samples in buffer":u32, "Lockin out"=w101:dbl[][])  [unwired: 6 in, 1 out]
      n26 = Index Array(array=w101, index (row) #1=0 ("index"), index (row) #2=1 ("length")) -> (element #1=w103:dbl[], element #2=w102:dbl[])  [unwired: 2 in]
      n27 = Re/Im To Complex(1:w102, 2:w103) -> (0:w110:cdb[])
      n28 = call "single sweep - upload freq window.vi"("first time ?"=w96, "timeout"=w114, "error in (no error)"=w112, "F-window array"=w95, "task in"=w120, "RUS settings"=w119) -> ("error out"=w111:errorcluster, "task out"=w115:refnum<k21>, "RUS settings out"=w118:T14)  [unwired: 1 in, 2 out]
      n29 = Not(x=w96) -> (.not. x?=w97:bool)
      n30 = call "single sweep - upload freq window.vi"("first time ?"=w97, "timeout"=w114, "error in (no error)"=w111, "F-window array"=w94, "task in"=w115, "RUS settings"=w118) -> ("error out"=w99:errorcluster, "task out"=w116:refnum<k21>, "RUS settings out"=w117:T14)  [unwired: 1 in, 2 out]
      n31 = Merge Errors(w100, w99) -> (w113:errorcluster)
    }
    frame "Pitaya" {
      n32 = Unbundle By Name(w133) -> ("RP Transeiver"=w132:refnum<class "RP Transceiver.lvclass">)
      n33 = Build Array (concatenate)(w135, w123) -> (w134:dbl[])
      n34 = Array Size(array=w123) -> (size(s)=w122:i32)
      n35 = call-dynamic "Transmit Lockin Data.vi"("error in (no error)"=w131, "Data"=w134, "RP Transceiver in"=w132) -> ("error out"=w129:errorcluster, "RP Transceiver out"=w130:refnum<class "RP Transceiver.lvclass">)  [unwired: 6 in, 1 out]
      n36 = call-dynamic "Recieve Lockin Data.vi"("error in (no error)"=w129, "Points to read"=w122, "RP Lockin in"=w130) -> ("error out"=w125:errorcluster, "Volatge X out"=w128:dbl[], "Frequency out"=w124:dbl[], "RP Lockin out"=w126:refnum<class "RP Transceiver.lvclass">)  [unwired: 2 in, 3 out]
      n37 = Bundle By Name(cluster=w133, "RP Transeiver"=w126) -> (w127:T14)
    }
  }
  n38 = property on="progress (sec)" class="Slide (strict)"("Scale.Maximum"=w37, "Scale.Minimum"=0.0 ("Data Entry Limits:Minimum")) -> ()  [unwired: 2 in, 2 out]
  n39 = Divide(x=w34, y=w33) -> (x/y=w85:dbl)
  n40 = register-events(w51, w45) -> (reference out=w53:refnum<event-registration>)  [unwired: 2 in, 1 out]
  n41 = Round Toward +Infinity(x=w85) -> (ceil(x): smallest int >= x=w79:dbl)
  n42 = Create User Event(user event datatype=w8) -> (user event=w4:refnum<user-event>)  [unwired: 1 in, 1 out]
  n43 = To Long Integer(number=w79) -> (32bit integer=w66:i32)
  n44 = Decrement(x=w66) -> (x-1=w75:i32)
  n45 = Tick Count (ms)() -> (millisecond timer value=w86:u32)
  n46 = Initialize Array(0.0 ("Numeric"), w34) -> (w47:dbl[])
  n47 = register-events(w4) -> (reference out=w7:refnum<event-registration>)  [unwired: 2 in, 1 out]
  n48 = call "next chunk - V4.vi"("next chunk action"=w14, "x + iy"=w25, "chunks"=w30) -> ("chunks out"=w29:T13, "F Array out"=w27:dbl[])  [unwired: 5 in, 2 out]
  n49 = Initialize Array(cdb 0.0+0.0i ("Numeric"), w34) -> (w77:cdb[])
  n50 = Add(x="Graph update rate, ms", y=w86) -> (x+y=w59:u32)
  n51 = local write "Progress, %"(u8 0 ("Progress")) -> ()
  n52 = while {
    tunnel: w7 -> [w141]
    tunnel: w6 -> [w140]
    tunnel: w4 -> [w139]
    tunnel: w5 -> [w138]
    stop <- w137 stop-if-true
    n53 = Wait (ms)(milliseconds to wait=u32 11) -> ()  [unwired: 1 out]
    n54 = event shown="[3] \"Plot:complex plane\": Cursor Move" {
      selector: w141 -> [_ _ _ _ _]
      dyn-events: _ -> [_ _ _ _ _]
      timeout: _ -> [_ _ _ _ _]
      tunnel: w140 -> [_ w145 _ _ w246]
      tunnel: w139 -> [_ w144 w240 w242 _]
      tunnel: w138 -> [_ _ _ _ w244]
      tunnel: [_ w143 _ _ _] -> w137
      event Timeout {
        n55 = event-data() -> ()  [unwired: 1 in, 2 out]
      }
      event User Event {
        n56 = event-data() -> ("action"=w146:string)  [unwired: 1 in]
        n57 = case shown="\"draw circle\"" w146 {
          tunnel: w145 -> [_ w163 _ w168 _ w193]
          tunnel: w144 -> [_ w161 _ _ _ _]
          tunnel: [FALSE FALSE TRUE FALSE FALSE FALSE] -> w143
          frame "False", Default {
          }
          frame "scale gauge changed" {
            n58 = local read "complex plane scale gauge"() -> (w152:dbl)
            n59 = local read "last data"() -> (w148:cdb[])
            n60 = Add Array Elements(numeric array=w148) -> (sum=w159:cdb)
            n61 = Array Size(array=w148) -> (size(s)=w158:i32)
            n62 = Divide(x=w159, y=w158) -> (x/y=w157:cdb)
            n63 = Complex To Re/Im(x + iy=w157) -> (x=w156:dbl, y=w153:dbl)
            n64 = Negate(x=w152) -> (-x=w151:dbl)
            n65 = Add(x=w156, y=w152) -> (x+y=w155:dbl)
            n66 = Add(x=w156, y=w151) -> (x+y=w154:dbl)
            n67 = Generate User Event(user event=w161, event data cluster="draw circle" ("event data")) -> ()  [unwired: 2 in, 2 out]
            n68 = Add(x=w153, y=w152) -> (x+y=w150:dbl)
            n69 = Add(x=w153, y=w151) -> (x+y=w149:dbl)
            n70 = property on="Property Node" class="XYGraph (strict)"(reference=w163, "XScale.Maximum"=w155, "XScale.Minimum"=w154, "YScale.Maximum"=w150, "YScale.Minimum"=w149) -> ()  [unwired: 1 in, 2 out]
          }
          frame "stop" {
          }
          frame "draw circle" {
            w180 = cursor_action."range" ("cursor action")
            n71 = call "replace cursor - plot ref - V2.vi"("Plot ref in"=w168, "cursor index"=0, "cursor action"=w180) -> ("read X"=w178:dbl, "read Y"=w177:dbl)  [unwired: 14 in, 1 out]
            n72 = call "replace cursor - plot ref - V2.vi"("Plot ref in"=w168, "cursor index"=1, "cursor action"=w180) -> ("read X"=w175:dbl, "read Y"=w174:dbl)  [unwired: 14 in, 1 out]
            n73 = Re/Im To Complex(1:w177, 2:w178) -> (0:w176:cdb)
            n74 = Re/Im To Complex(1:w174, 2:w175) -> (0:w173:cdb)
            n75 = Bundle By Name(cluster=T17 {"z (-pi/2)"=-1.0311345636926572+0.5736824521422934i, "z(inf)"=-0.5200164984937075+1.0975277942502903i, "z (pi/2)"=-1.0311345636926572+0.5736824521422934i, "z center"=-0.5136528600391839+0.580046090596817i, "z(0)"=-0.5200164984937075+1.0975277942502903i, "radius"=-1.0311345636926572} ("circle corners in"), "z center"=w176, "z(0)"=w173) -> (w167:T17)
            n76 = call "peak -- four corner circle transformation logic.vi"("4 corner circle transformation"=four-corner_circle_transformation."z(c) z(zero)", "circle corners in"=w167) -> ("circle corners out"=w172:T17)  [unwired: 8 in, 1 out]
            n77 = call "draw - 4 corner circle.vi"("4corners"=w172) -> ("line two"=→"line two":cluster{dbl[], dbl[]}, "line one"=→"line one":cluster{dbl[], dbl[]}, "circle"=→"circle":cluster{dbl[], dbl[]})  [unwired: 8 in]
          }
          frame "fit lorentzian" {
            n78 = case shown="False" FALSE {
              frame False {
              }
              frame True {
                n79 = call "filter - complex - four.vi"() -> ()  [unwired: 12 in, 8 out]
                n80 = call "peak -- PM find lorenzian - V2.vi"() -> ()  [unwired: 12 in, 4 out]
                n81 = call "peak -- four corner circle transformation logic.vi"("4 corner circle transformation"=four-corner_circle_transformation."calculate lorentzian") -> ()  [unwired: 9 in, 2 out]
              }
            }
          }
          frame "plot all" {
            # "last 1 sec segment"
            n82 = local read "#data points so far"() -> (w189:i32)
            n83 = local read "complex data"() -> (w190:cdb[])
            n84 = case shown="\"No\"" "Subtract a circle?" {
              tunnel: w193 -> [w231 _]
              tunnel: [w222 w239] -> w192
              tunnel: w190 -> [w221 w239]
              frame "Yes", Default {
                w236 = cursor_action."range" ("cursor action")
                n85 = call "replace cursor - plot ref - V2.vi"("Plot ref in"=w231, "cursor index"=0, "cursor action"=w236) -> ("read X"=w235:dbl, "read Y"=w234:dbl)  [unwired: 14 in, 1 out]
                n86 = call "replace cursor - plot ref - V2.vi"("Plot ref in"=w231, "cursor index"=1, "cursor action"=w236) -> ("read X"=w233:dbl, "read Y"=w232:dbl)  [unwired: 14 in, 1 out]
                n87 = Re/Im To Complex(1:w234, 2:w235) -> (0:w228:cdb)
                n88 = Re/Im To Complex(1:w232, 2:w233) -> (0:w230:cdb)
                n89 = Subtract(x=w230, y=w228) -> (x-y=w229:cdb)
                n90 = Subtract(x=w221, y=w228) -> (x-y=w227:cdb[])
                n91 = Complex To Polar(r * e^(i*theta)=w229) -> (r=w225:dbl)  [unwired: 1 out]
                n92 = Complex To Polar(r * e^(i*theta)=w227) -> (r=w226:dbl[])  [unwired: 1 out]
                n93 = Divide(x=w226, y=w225) -> (x/y=w224:dbl[])
                n94 = Divide(x=w221, y=w224) -> (x/y=w223:cdb[])
                n95 = Subtract(x=w221, y=w223) -> (x-y=w222:cdb[])
              }
              frame "No" {
              }
            }
            n96 = local read "chunks"() -> (w198:T13)
            n97 = Unbundle By Name(w198) -> ("update rate (Hz)"=w200:dbl)
            n98 = Multiply(x="highlight last # sec", y=w200) -> (x*y=w201:dbl)
            n99 = Round Toward -Infinity(1:w201) -> (0:w202:dbl)
            n100 = To Long Integer(number=w202) -> (32bit integer=w196:i32)
            n101 = Subtract(x=w189, y=w196) -> (x-y=w195:i32)
            n102 = Array Subset(array=w190, index=w195, length=w196) -> (w209:cdb[])
            n103 = local read "frequency"() -> (w197:dbl[])
            n104 = Array Subset(array=w192, length=w189) -> (w207:cdb[])  [unwired: 1 in]
            n105 = Array Subset(array=w190, length=w189) -> (w191:cdb[])  [unwired: 1 in]
            n106 = Complex To Re/Im(x + iy=w209) -> (x=w210:dbl[], y=w211:dbl[])
            n107 = Complex To Re/Im(x + iy=w207) -> (x=w215:dbl[], y=w216:dbl[])
            n108 = Complex To Re/Im(x + iy=w191) -> (x=w188:dbl[], y=w187:dbl[])
            n109 = Divide(x=w197, y=1000 ("dimension size")) -> (x/y=w213:dbl[])
            n110 = local read "line one"() -> (w219:cluster{dbl[], dbl[]})
            n111 = local read "circle"() -> (w218:cluster{dbl[], dbl[]})
            n112 = local read "line two"() -> (w220:cluster{dbl[], dbl[]})
            n113 = local read "fancy lines"() -> (w217:cluster{dbl[], dbl[]}[])
            n114 = Bundle(w213, w215) -> (w203:cluster{dbl[], dbl[]})  [unwired: 1 out]
            n115 = Bundle(w213, w216) -> (w205:cluster{dbl[], dbl[]})  [unwired: 1 out]
            n116 = Bundle(w188, w187) -> (w208:cluster{dbl[], dbl[]})  [unwired: 1 out]
            n117 = Bundle(w210, w211) -> (w212:cluster{dbl[], dbl[]})  [unwired: 1 out]
            n118 = Build Array (concatenate)(w203, w205, w217) -> (→"Plot:response":cluster{dbl[], dbl[]}[])
            n119 = Build Array(w208, w212, w218, w219, w220) -> (→"Plot:complex plane":cluster{dbl[], dbl[]}[])
          }
        }
      }
      event "complex plane scale gauge": Value Change {
        n120 = event-data() -> ()  [unwired: 1 in, 1 out]
        n121 = Generate User Event(user event=w240, event data cluster="scale gauge changed" ("event data")) -> ()  [unwired: 2 in, 2 out]
      }
      event "Plot:complex plane": Cursor Move {
        n122 = event-data() -> ()  [unwired: 1 in, 5 out]
        n123 = Generate User Event(user event=w242, event data cluster="draw circle" ("event data")) -> ()  [unwired: 2 in, 2 out]
      }
      event "show plot pallets": Value Change {
        n124 = event-data() -> ("NewVal"=w245:bool)  [unwired: 1 in]
        n125 = property on="Property Node" class="XYGraph (strict)"(reference=w246, "ScaleLegendVis"=w245, "Palette Visible"=w245, "Legend Visible"=w245) -> ()  [unwired: 1 in, 2 out]
        n126 = property on="Property Node" class="XYGraph (strict)"(reference=w244, "ScaleLegendVis"=w245, "Palette Visible"=w245, "Legend Visible"=w245) -> ()  [unwired: 1 in, 2 out]
      }
    }
  }
  n127 = while {
    tunnel: w53 -> [w259]
    shift-right: [w257] -> w72
    shift-left: w77 -> [w256]
    shift-right: [w253] -> _
    shift-left: w59 -> [w255]
    tunnel: "Graph update rate, ms" -> [w254]
    shift-right: [w251] -> w42
    shift-left: 0 ("disabled index (col)") -> [w252]
    shift-right: [w249] -> w43
    shift-left: w47 -> [w250]
    tunnel: w6 -> [w248]
    tunnel: w4 -> [w247]
    stop <- w258 stop-if-true
    # "dispatch loop"
    n128 = event shown="[1] <New data>: User Event" {
      selector: w259 -> [_ _ _]
      dyn-events: _ -> [_ _ _]
      timeout: _ -> [_ _ _]
      tunnel: [_ _ TRUE] -> w258
      tunnel: [w263 w281 w298] -> w257
      tunnel: w256 -> [w263 w282 w298]
      tunnel: w255 -> [w262 w278 w297]
      tunnel: w254 -> [_ w276 _]
      tunnel: [w262 w284 w297] -> w253
      tunnel: w252 -> [w261 w270 w296]
      tunnel: [w261 w267 w296] -> w251
      tunnel: w250 -> [w260 w272 w295]
      tunnel: [w260 w271 w295] -> w249
      tunnel: w248 -> [_ _ _]
      tunnel: w247 -> [_ w264 w293]
      event Timeout {
        n129 = event-data() -> ()  [unwired: 3 out]
      }
      event User Event {
        # "complex data"
        # "frequency"
        # "Plot data"
        # "New data arrives as a 2D complex array. Two rows are: \n1. frequency (as a complex number) ........... \n2. complex response .............."
        # "Insert new data"
        n130 = event-data() -> ("New data"=w275:cdb[][])  [unwired: 1 out]
        n131 = Tick Count (ms)() -> (millisecond timer value=w277:u32)
        n132 = Index Array(array=w275, index (row) #1=0 ("disabled index (col)"), index (row) #2=1 ("disabled index (col)")) -> (element #1=w269:cdb[], element #2=w266:cdb[])  [unwired: 2 in]
        n133 = Complex To Re/Im(x + iy=w269) -> (x=w268:dbl[])  [unwired: 1 out]
        n134 = Replace Array Subset(array=w272, new element=w268, index=w270) -> (w271:dbl[])
        "frequency" <- w271
        n135 = Replace Array Subset(array=w282, new element=w266, index=w270) -> (w281:cdb[])
        "complex data" <- w281
        n136 = Array Size(array=w266) -> (size(s)=w265:i32)
        n137 = Less?(x=w278, y=w277) -> (x < y?=w280:bool)
        n138 = Add(x=w265, y=w270) -> (x+y=w267:i32)
        "#data points so far" <- w267
        n139 = And(x=w280, y="Plot when running") -> (x .and. y?=w283:bool)
        n140 = case shown="True" w283 {
          tunnel: w281 -> [_ _]
          tunnel: w277 -> [_ w289]
          tunnel: [w285 w288] -> w284
          tunnel: w278 -> [w285 _]
          tunnel: w271 -> [_ _]
          tunnel: w276 -> [_ w290]
          tunnel: w264 -> [_ w286]
          frame False {
          }
          frame True {
            n141 = Add(x=w290, y=w289) -> (x+y=w288:u32)
            n142 = Generate User Event(user event=w286, event data cluster="plot all" ("event data")) -> ()  [unwired: 2 in, 2 out]
          }
        }
      }
      event User Event {
        n143 = event-data() -> ()  [unwired: 2 out]
        n144 = Generate User Event(user event=w293, event data cluster="plot all" ("event data")) -> (user event out=w292:refnum<user-event>)  [unwired: 2 in, 1 out]
        n145 = Generate User Event(user event=w292, event data cluster="stop" ("event data")) -> ()  [unwired: 2 in, 2 out]
      }
    }
  }
  n146 = for {
    N: w66 -> [w344]
    tunnel: w33 -> [w346]
    tunnel: [w323] -> w78
    tunnel: w75 -> [w340]
    tunnel: w34 -> [w347]
    tunnel: ["stop"] -> w71
    shift-right: [w336] -> w44
    shift-left: w32 -> [w337]
    shift-right: [w331] -> w55
    shift-left: _ -> [_]
    shift-right: [w311] -> _
    shift-left: w31 -> [w333]
    shift-right: [w313] -> w26
    shift-left: w28 -> [w314]
    shift-right: [w335] -> _
    shift-left: w27 -> [w315]
    shift-right: [w326] -> _
    shift-left: w29 -> [w334]
    shift-right: [w332] -> w54
    shift-left: _ -> [_]
    tunnel: w51 -> [w330]
    shift-right: [w318] -> _
    shift-left: _ -> [_]
    shift-right: [w317] -> _
    shift-left: _ -> [w319]
    shift-right: [w316] -> _
    shift-left: w25 -> [w312]
    shift-left: w24 -> [w301]
    shift-left: w13 -> [w310]
    tunnel: w14 -> [w309]
    shift-right: [w300] -> _
    shift-left: w2 -> [w303]
    tunnel: w1 -> [w302]
    i -> [w323]
    stop <- w349 stop-if-true
    (unwired) next_chunk_--_action."next chunk - peaks are known" ("next chunk action")
    (unwired) 1 ("length")
    (unwired) 1 ("index")
    # "build 2D array { freq; complex response}"
    # "Data aquisition loop"
    n147 = Less?(x=w340, y=w323) -> (x < y?=w348:bool)
    n148 = Equal To 0?(x=w323) -> ()  [unwired: 1 out]
    n149 = Divide(x=w323, y=w344) -> (x/y=w343:dbl)
    n150 = case shown="True" w348 {
      tunnel: w347 -> [_ w394]
      tunnel: w346 -> [_ w389]
      tunnel: w323 -> [_ w388]
      tunnel: w337 -> [w387 w392]
      tunnel: [w387 w390] -> w345
      frame False {
      }
      frame True {
        # "Round down  last read"
        n151 = Multiply(x=w389, y=w388) -> (x*y=w393:i32)
        n152 = Subtract(x=w394, y=w393) -> (x-y=w391:i32)
        n153 = Bundle By Name(cluster=w392, "Samples per read"=w391) -> (w390:T14)
      }
    }
    n154 = case shown="\"Pitaya\"" w302 {
      tunnel: w345 -> [_ w386]
      tunnel: w337 -> [w359 w385]
      tunnel: [w358 w384] -> w336
      tunnel: w333 -> [w357 w383]
      tunnel: [w352 w382] -> w332
      tunnel: [w352 w381] -> w331
      tunnel: [w356 w372] -> w316
      tunnel: w315 -> [w351 w371]
      tunnel: w314 -> [w355 w370]
      tunnel: [w354 w369] -> w313
      tunnel: [w357 w367] -> w311
      tunnel: w301 -> [_ w364]
      tunnel: [w353 w364] -> w300
      frame "Pitaya" {
        w352 = u32 0 ("DO write time")
        n155 = Unbundle By Name(w359) -> ("RP Transeiver"=w363:refnum<class "RP Transceiver.lvclass">)
        n156 = call-dynamic "Transmit Lockin Data.vi"("error in (no error)"=w355, "Data"=w351, "RP Transceiver in"=w363) -> ("error out"=w361:errorcluster, "RP Transceiver out"=w362:refnum<class "RP Transceiver.lvclass">)  [unwired: 6 in, 1 out]
        n157 = Array Size(array=w351) -> (size(s)=w350:i32)
        n158 = call-dynamic "Recieve Lockin Data.vi"("error in (no error)"=w361, "Points to read"=w350, "RP Lockin in"=w362) -> ("error out"=w354:errorcluster, "Volatge X out"=w356:dbl[], "Frequency out"=w353:dbl[], "RP Lockin out"=w360:refnum<class "RP Transceiver.lvclass">)  [unwired: 2 in, 3 out]
        n159 = Bundle By Name(cluster=w359, "RP Transeiver"=w360) -> (w358:T14)
      }
      frame "NI-DAQ", Default {
        w365 = 0.01  # timeout
        w373 = FALSE  # first time ?
        w380 = FALSE  # first time ?
        n160 = call "single sweep - upload freq window.vi"("first time ?"=w380, "timeout"=w365, "error in (no error)"=w370, "F-window array"=w371, "task in"=w383, "RUS settings"=w385) -> ("error out"=w366:errorcluster, "task out"=w367:refnum<k21>, "RUS settings out"=w384:T14, "DO array  making time"=w381:u32, "DO write time"=w382:u32)  [unwired: 1 in]
        n161 = call "NI-DAQ RUS Lockin.vi"("Init?"=w373, "error in (no error)"=w370, "RUS settings"=w386) -> ("error out"=w368:errorcluster, "AvailSampPerChan"=w374:u32, "Lockin out"=w379:dbl[][])  [unwired: 5 in, 1 out]
        n162 = local write "Samples in buffer"(w374) -> ()
        n163 = Merge Errors(w368, w366) -> (w369:errorcluster)
        n164 = Index Array(array=w379, index (row) #1=0 ("index"), index (row) #2=1 ("length")) -> (element #1=w376:dbl[], element #2=w375:dbl[])  [unwired: 2 in]
        n165 = Re/Im To Complex(1:w375, 2:w376) -> (0:w372:cdb[])
      }
    }
    "last data" <- w316
    n166 = Multiply(x=w343, y=100.0) -> (x*y=→"Progress, %":dbl)
    n167 = Re/Im To Complex(1:0.0, 2:w303) -> (0:w328:cdb[])
    n168 = Build Array(w328, w312) -> (w327:cdb[][])
    n169 = Generate User Event(user event=w330, event data cluster=w327) -> ()  [unwired: 2 in, 2 out]
    n170 = Unbundle By Name(w345) -> ()  [unwired: 2 out]
    n171 = call "next chunk - V4.vi"("next chunk action"=w309, "x + iy"=w312, "chunks"=w334, "F Array in"=w310) -> ("chunks out"=w308:T13, "F Array out"=w335:dbl[], "fancy lines"=→"fancy lines":cluster{dbl[], dbl[]}[], "fancy circles"=→"fancy circles":cluster{dbl[], dbl[]}[])  [unwired: 4 in]
    n172 = local read "adaptive state"() -> (w325:T9)
    n173 = Unbundle By Name(w308) -> ("adaptive parameters.peaks are known -- parameters.near omega (kHz)"=→"near omega (kHz)":dbl, "adaptive parameters.peaks are known -- parameters.near gamma (kHz)"=→"near gamma (kHz)":dbl)
    n174 = Tick Count (ms)() -> (millisecond timer value=w322:u32)
    n175 = Bundle By Name(cluster=w308, "adaptive parameters"=w325) -> (w326:T13)
    n176 = Divide(x=w322, y=u32 1000) -> (x/y=w318:dbl)
    n177 = Equal To 0?(x=w323) -> (x = 0?=w320:bool)
    n178 = Select(t=w318, s=w320, f=w319) -> (s? t:f=w317:dbl)
    n179 = Unbundle By Name(w313) -> ("status"=w338:bool)
    n180 = Subtract(x=w318, y=w317) -> (x-y=w324:dbl)
    n181 = local write "progress (sec)"(w324) -> ()
    n182 = local write "chunks"(w326) -> ()
    n183 = Compound Arithmetic op=OR("stop", w338) -> (w349:bool)
  }
  "Loop counter" <- w78
  "DO array  making time" <- w55
  "DO write time, ms" <- w54
  n184 = Increment(x=w78) -> (x+1=w74:i32)
  n185 = Divide(x=w74, y=w79) -> (x/y=w82:dbl)
  n186 = Multiply(x=w82, y=100.0) -> (x*y=w80:dbl)
  n187 = local write "Progress, %"(w80) -> ()
  n188 = disable-structure shown="Disabled" {
    frame Disabled {
      n189 = Unbundle By Name() -> ("Lockin mode"=w395:enum16{"SRS", "NI-DAQ"})  [unwired: 1 in]
      n190 = case shown="\"NI-DAQ\"" w395 {
        tunnel: [_ w397] -> _
        tunnel: [_ w396] -> _
        frame "SRS", Default {
        }
        frame "NI-DAQ" {
          # "Download freq array"
          n191 = call "ProgramFreqBulk.vi"() -> ("error out"=w397:errorcluster, "RUS settings out"=w396:T14)  [unwired: 5 in, 5 out]
        }
      }
    }
    frame Enabled {
    }
  }
  n192 = Unbundle By Name("sweep settings") -> ("Zero signal?"=w10:bool, "save freq units"=w9:enum16{"kHz", "Hz"}, "Bypass error dialog"=w11:bool)
  n193 = Array Subset(array=w43, length=w42) -> (w35:dbl[])  [unwired: 1 in]
  n194 = Array Subset(array=w72, length=w42) -> (w46:cdb[])  [unwired: 1 in]
  n195 = call "single sweep - rus clean up.vi"("Zero amplitude at the end"=w10, "Stop user event"=w45, "error in (no error)"=w26, "RUS settings"=w44) -> ("error out"=w67:errorcluster, "STD status byte"=→"STD status byte":u8, "Error status byte\n(bit 5 - FAST aborted)"=→"Error status byte\n(bit 5 - FAST aborted)":u8, "RUS settings out"=w62:T14)  [unwired: 4 in]
  n196 = Not(x=w71) -> (.not. x?=w60:bool)
  n197 = disable-structure shown="Enabled" {
    disable-tunnel: w46 -> [w407 _]
    disable-tunnel: w35 -> [w400 _]
    frame Disabled {
      n198 = Complex To Re/Im(x + iy=w407) -> (x=w406:dbl[], y=w405:dbl[])
      n199 = disable-structure shown="Enabled" {
        disable-tunnel: w405 -> [w415 w417]
        disable-tunnel: w406 -> [w414 w416]
        disable-tunnel: [w413 w416] -> w403
        disable-tunnel: [w412 w417] -> w402
        disable-tunnel: _ -> [w411 _]
        frame Disabled {
          n200 = call "Rotate Lockin Phase.vi"("Phase"=w411, "Array Y in"=w415, "Array X in"=w414) -> ("Array Y out"=w412:dbl[], "Array X out"=w413:dbl[])  [unwired: 7 out]
        }
        frame Enabled {
        }
      }
      n201 = Divide(x=w400, y=1000 ("dimension size")) -> (x/y=w399:dbl[])
      n202 = Bundle(w403, w402) -> (w404:cluster{dbl[], dbl[]})  [unwired: 1 out]
      n203 = Bundle(w399, w403) -> (w410:cluster{dbl[], dbl[]})  [unwired: 1 out]
      n204 = Bundle(w399, w402) -> (w409:cluster{dbl[], dbl[]})  [unwired: 1 out]
      n205 = Build Array(w410, w409) -> (w408:cluster{dbl[], dbl[]}[])
      n206 = Build Array(w404) -> (w401:cluster{dbl[], dbl[]}[])
      n207 = local write "Plot:complex plane"(w401) -> ()
      n208 = local write "Plot:response"(w408) -> ()
    }
    frame Enabled {
    }
  }
  n209 = case shown="True" w60 {
    tunnel: w67 -> [w418 w425]
    tunnel: [w418 w423] -> w84
    tunnel: w46 -> [_ w420]
    tunnel: w62 -> [_ w422]
    tunnel: w35 -> [_ w421]
    tunnel: w9 -> [_ w419]
    frame False {
    }
    frame True {
      n210 = call "single sweep - save rus data.vi"("save freq units"=w419, "error in (no error)"=w425, "rus response"=w420, "F Array"=w421, "RUS settings"=w422) -> ("error out"=w423:errorcluster, "Actual file path"=→"Actual file path":path)  [unwired: 5 in]
    }
  }
  n211 = disable-structure shown="Disabled" {
    frame Disabled {
      n212 = while {
        shift-right: [w429] -> _
        shift-left: _ -> [w430]
        shift-right: [w428] -> _
        shift-left: _ -> [w431]
        tunnel: [w426] -> _
        stop <- TRUE stop-if-true
        n213 = property class="DAQmx Write"(reference=w430, error in=w431) -> (reference out=w429:refnum<k21>, error out=w428:errorcluster, "SpaceAvail"=w426)
      }
    }
    frame Enabled {
    }
  }
  n214 = case shown="False" w11 {
    tunnel: [w433 w435] -> w87
    tunnel: w84 -> [w432 w435]
    frame False {
      w434 = T20 3 items=["no dialog", "OK message", "continue or stop message", "OK message + warnings", "continue/stop + warnings"] ("type of dialog (OK msg:1)")
      n215 = call <vilib>:"General Error Handler.vi"("type of dialog (OK msg:1)"=w434, "error in (no error)"=w432) -> ("error out"=w433:errorcluster)  [unwired: 1 in, 12 out]
    }
    frame True {
    }
  }
  "error out" <- w87
